vi "Example - Subscribe.vi"() -> ()   [LabVIEW 2020, in "wamplv.lvlib"]
uses:
  wamplv.lvlib
  WAMP Client/WAMP Client.lvclass/WAMP Client.ctl
  <vilib>/Utility/error.llb/Error Cluster From Error Code.vi
  WAMP Client/WAMP Client.lvclass
panel:
  out "Topic":string
  out "ArgumentKw Payload":string
  out "Arguments Payload":string
  out "Event received on:":string
  in  "Subscription URI":string="test.topic"
  in  "Disconnect":bool caption="Publish Topic"
  in  "Realm":string="default_realm"
  in  "Router Address":string="ws://localhost:8080/"
  # "Example: publish"
  # "This example will subscribe to the given topic, and display the publication/sevents \nas they are received.\n\nThe router URI must a fully-formed URI: \n\ntcp://localhost:8080/ (RawSocket TCP)\ntcps://localhost:8080/ (RawSocket TCP with TLS/SSL)\nws://localhost:8080/ (WebScoket)\nws://localhost:8080/ws (WebScoket)\nwss://localhost:8080/ (WebSocket TCP with TLS/SSL)\n\nAlways disconnect by pressing the disconnect button, not by aborting the VI. Otherwise the \nWAMP session will conitinue in the background."
  # "Receied Event:"
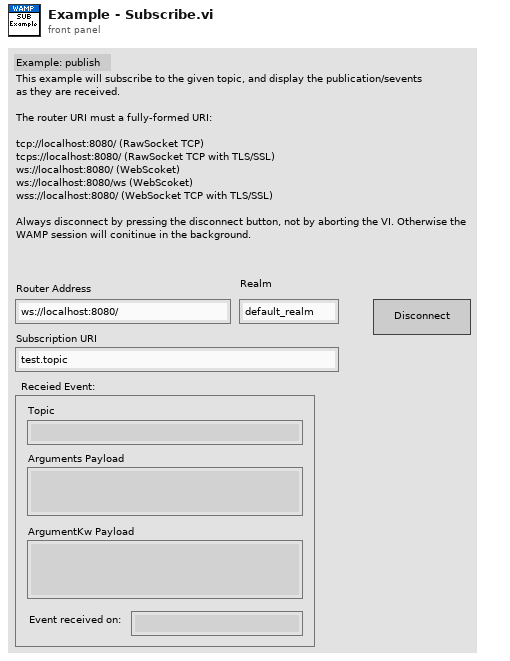
[diagram p1: front panel]
types:
  T1 = typedef "wamplv.lvlib/WAMP Client.lvclass/EVENT payload.ctl" = cluster{"Arguments Payload":string, "ArgumentKw Payload":string, "Topic":string}
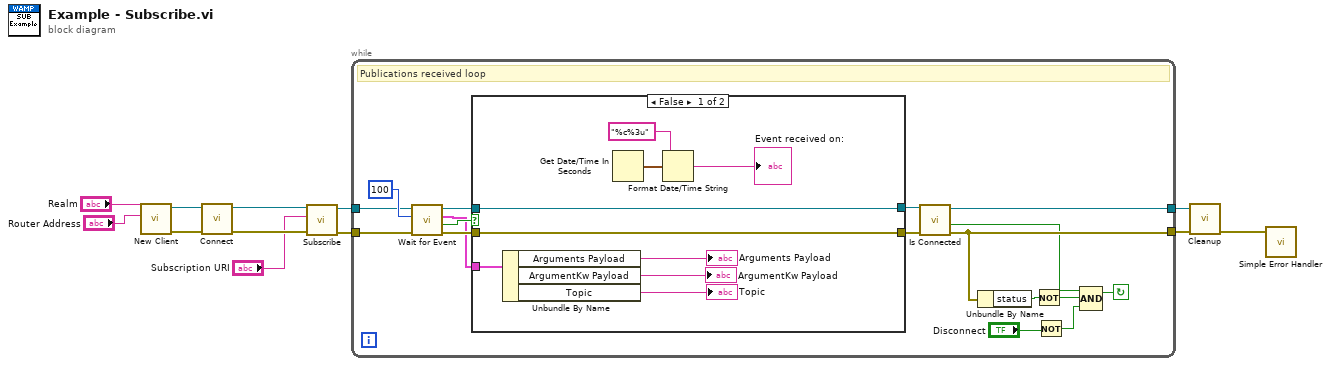
[diagram p0: block diagram]
diagram:
  n1 = call "New Client.vi"("Address"="Router Address", "Realm"="Realm") -> ("error out"=w8:errorcluster, "WAMP client out"=w10:refnum<class "WAMP Client.lvclass">)  [unwired: 8 in]
  n2 = call "Connect.vi"("error in"=w8, "WAMP Client in"=w10) -> ("error out"=w6:errorcluster, "WAMP Client out"=w7:refnum<class "WAMP Client.lvclass">)  [unwired: 8 in]
  n3 = call-dynamic "Subscribe.vi"("error in (no error)"=w6, "Topic"="Subscription URI", "WAMP Client in"=w7) -> ("error out"=w1:errorcluster, "WAMP Client out"=w2:refnum<class "WAMP Client.lvclass">)  [unwired: 4 in, 3 out]
  n4 = while {
    tunnel: [w20] -> w4
    tunnel: [w17] -> w3
    tunnel: w2 -> [w14]
    tunnel: w1 -> [w13]
    stop <- w18 continue-if-true
    # "Publications received loop"
    n5 = call "Wait for Event.vi"("error in (no error)"=w13, "timeout in ms (-1)"=100, "WAMP Client in"=w14) -> ("error out"=w26:errorcluster, "timed out?"=w28:bool, "WAMP Event"=w25:T1, "WAMP Client out"=w27:refnum<class "WAMP Client.lvclass">)  [unwired: 5 in]
    n6 = case shown="False" w28 {
      tunnel: w27 -> [w31 w39]
      tunnel: w26 -> [w30 w40]
      tunnel: w25 -> [w35 _]
      tunnel: [w31 w39] -> w24
      tunnel: [w30 w40] -> w23
      frame False {
        n7 = Unbundle By Name(w35) -> ("Arguments Payload"=→"Arguments Payload":string, "ArgumentKw Payload"=→"ArgumentKw Payload":string, "Topic"=→"Topic":string)
        n8 = Get Date/Time In Seconds() -> (seconds since 1Jan1904=w37:timestamp)
        n9 = Format Date/Time String(time format string (%c)="%c%3u", seconds (now)=w37) -> (date/time string=→"Event received on:":string)  [unwired: 1 in]
      }
      frame True {
      }
    }
    n10 = call "Is Connected.vi"("error in"=w23, "WAMP Client in"=w24) -> ("error out"=w20:errorcluster, "Is Connected?"=w19:bool, "WAMP Client out"=w17:refnum<class "WAMP Client.lvclass">)  [unwired: 7 in]
    n11 = Unbundle By Name(w20) -> ("status"=w22:bool)
    n12 = Not(x=w22) -> (.not. x?=w21:bool)
    n13 = Not(x="Disconnect") -> (.not. x?=w15:bool)
    n14 = Compound Arithmetic op=AND(w19, w21, w15) -> (w18:bool)
  }
  n15 = call-dynamic "Cleanup.vi"("error in"=w4, "WAMP Client in"=w3) -> ("error out"=w9:errorcluster)  [unwired: 8 in, 1 out]
  n16 = call <vilib>:"Simple Error Handler.vi"("error in (no error)"=w9) -> ()  [unwired: 4 in, 5 out]
